vi "新记录通知-服务器版.vi"() -> ()   [LabVIEW 2013]
uses:
  <vilib>/Utility/miscctls.llb/LVRowAndColumnTypeDef.ctl
  <vilib>/Utility/inputDevices.llb/mouseAcquire.vi
panel:
  in  "列表菜单":enum16{"预览", "忽略此条", "删除缓存文件", "复制到剪贴板"}(ring)
  out "点到行列-实时列表":T1 caption="单元格位置"
  in  "device ID":refnum<k1> caption="设备ID"
  in  "新记录":cluster{"新记录列表行":string[], "对应缓存文件":string}[](array[cluster])
  in  "报警记录列表":i32[](listbox)
  in  "忽略全部":bool
  in  "预览全部":bool
  # "* 双击单元格打开预览\n  右键菜单中查看更多选项，管理界面中查看更多记录"
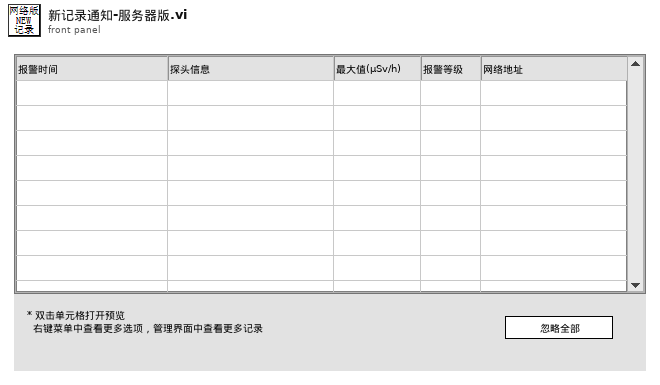
[diagram p1: front panel]
types:
  T1 = typedef "LVRowAndColumnTypeDef.ctl" = cluster{"Row":i32, "Column":i32}
  T2 = enum32{"Invalid", "Standard", "Closed", "Hidden", "Minimized", "Maximized"}
  T3 = typedef "LVPoint32TypeDef.ctl" = cluster{"Horizontal":i32, "Vertical":i32}
  T4 = cluster{"button 1":bool, "button 2":bool, "button 3":bool, "button 4":bool}
  T5 = cluster{"Shift":bool, "Ctrl":bool, "Alt":bool, "Cmd":bool, "Opt":bool}
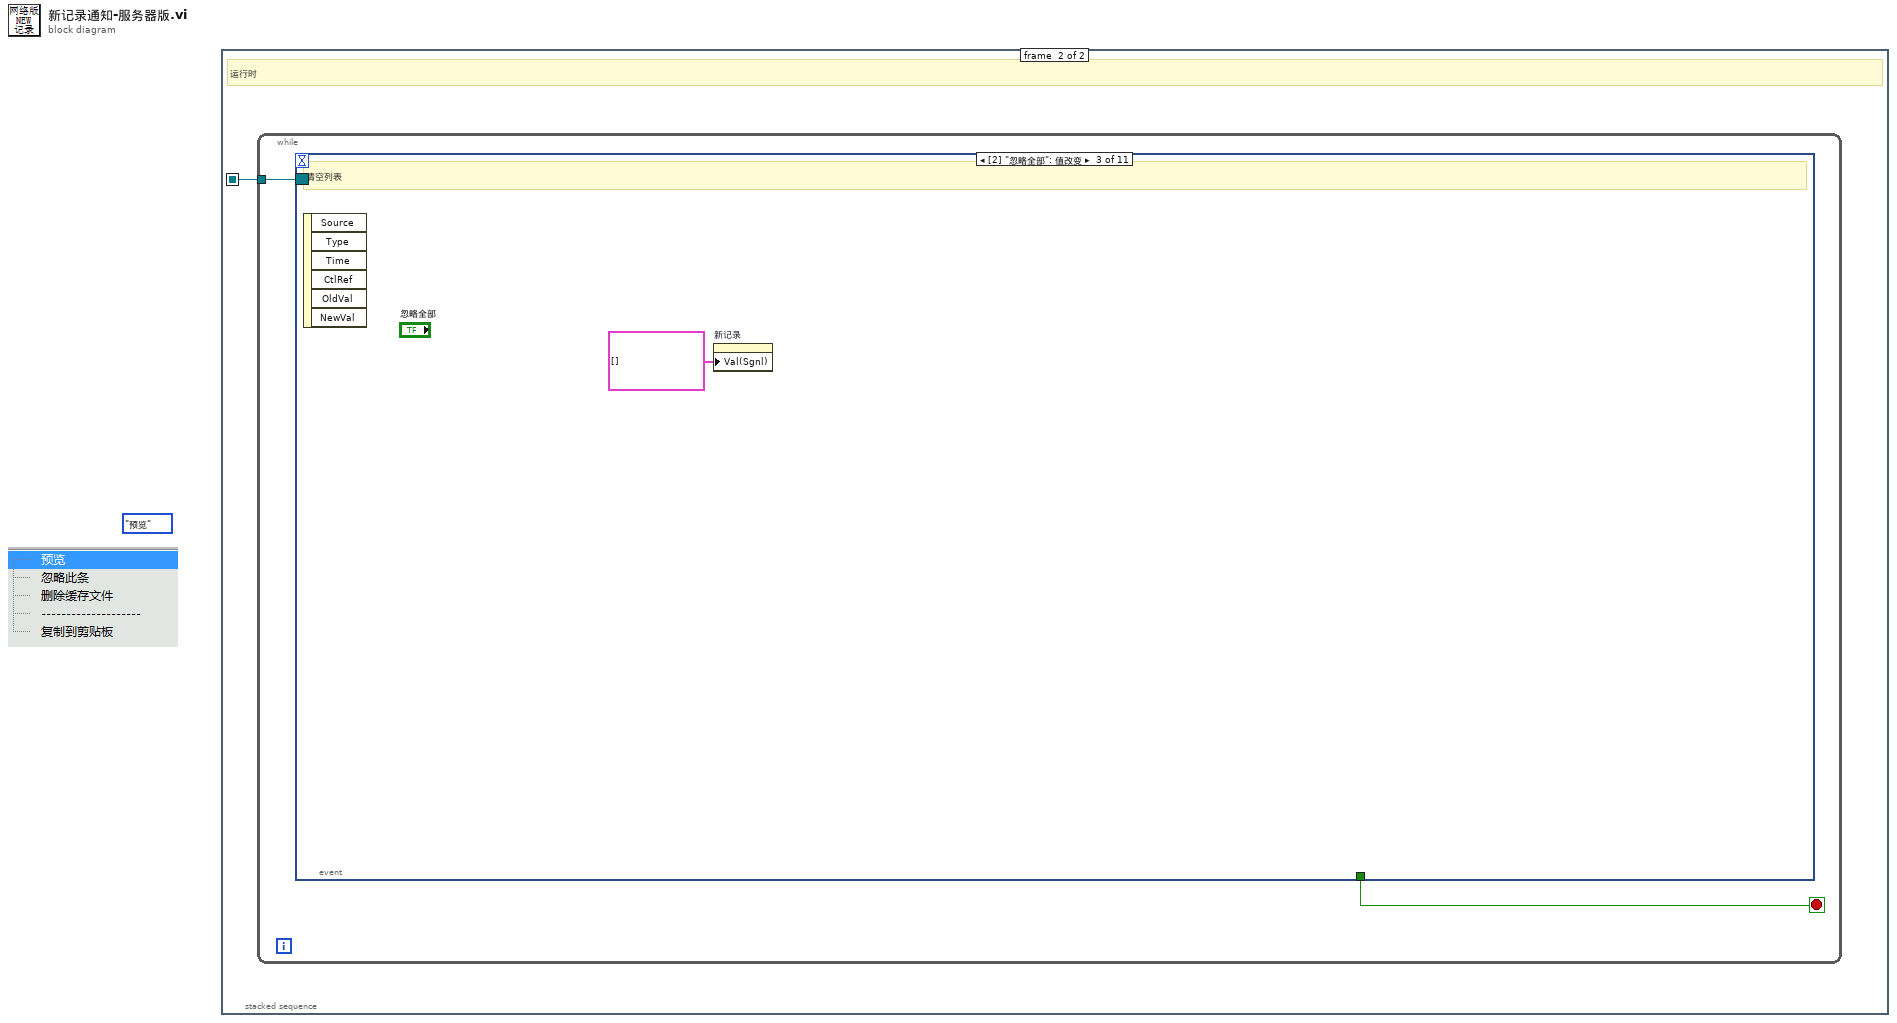
[diagram p0: block diagram]
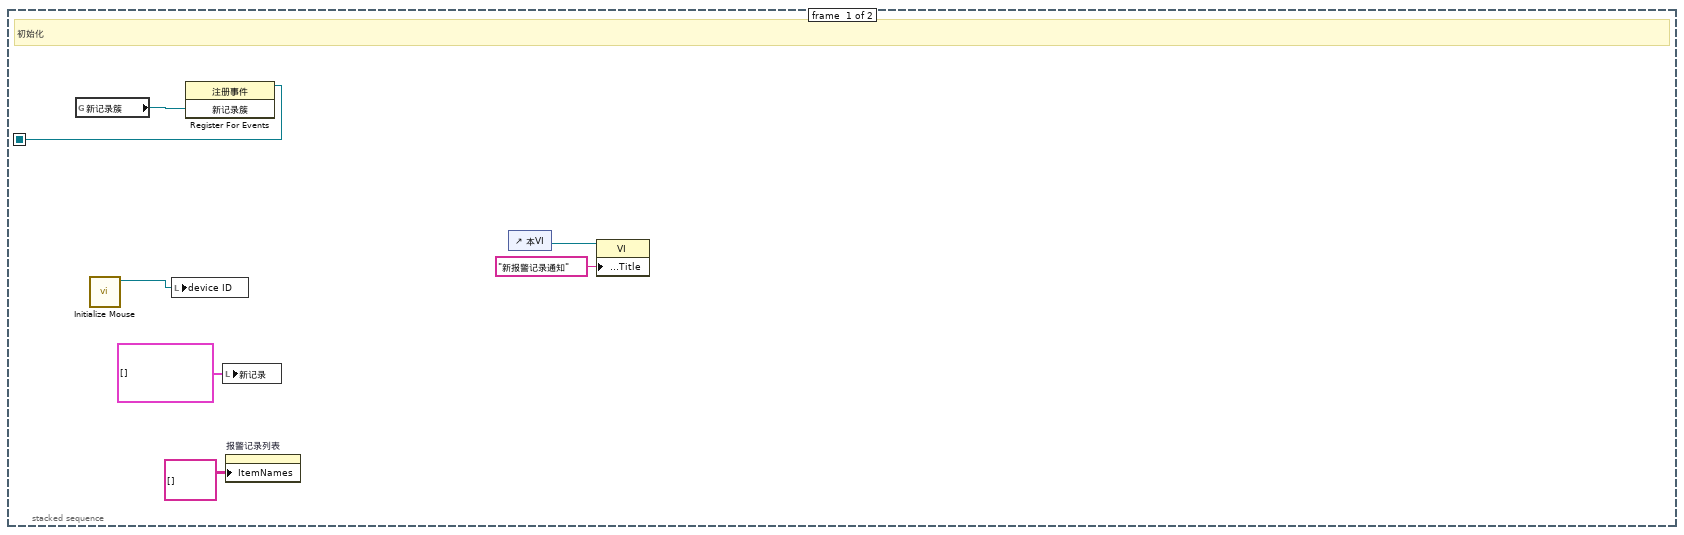
[diagram p2: hidden frame]
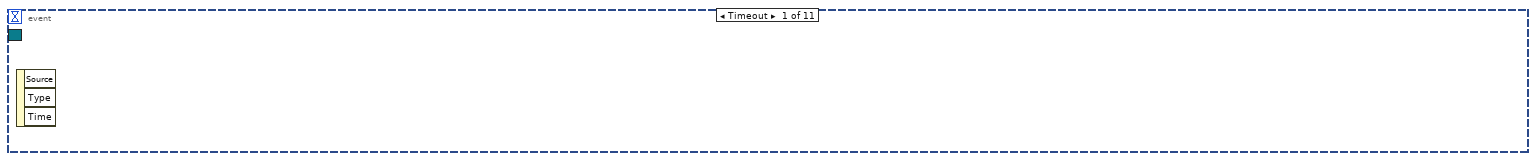
[diagram p3: hidden frame]
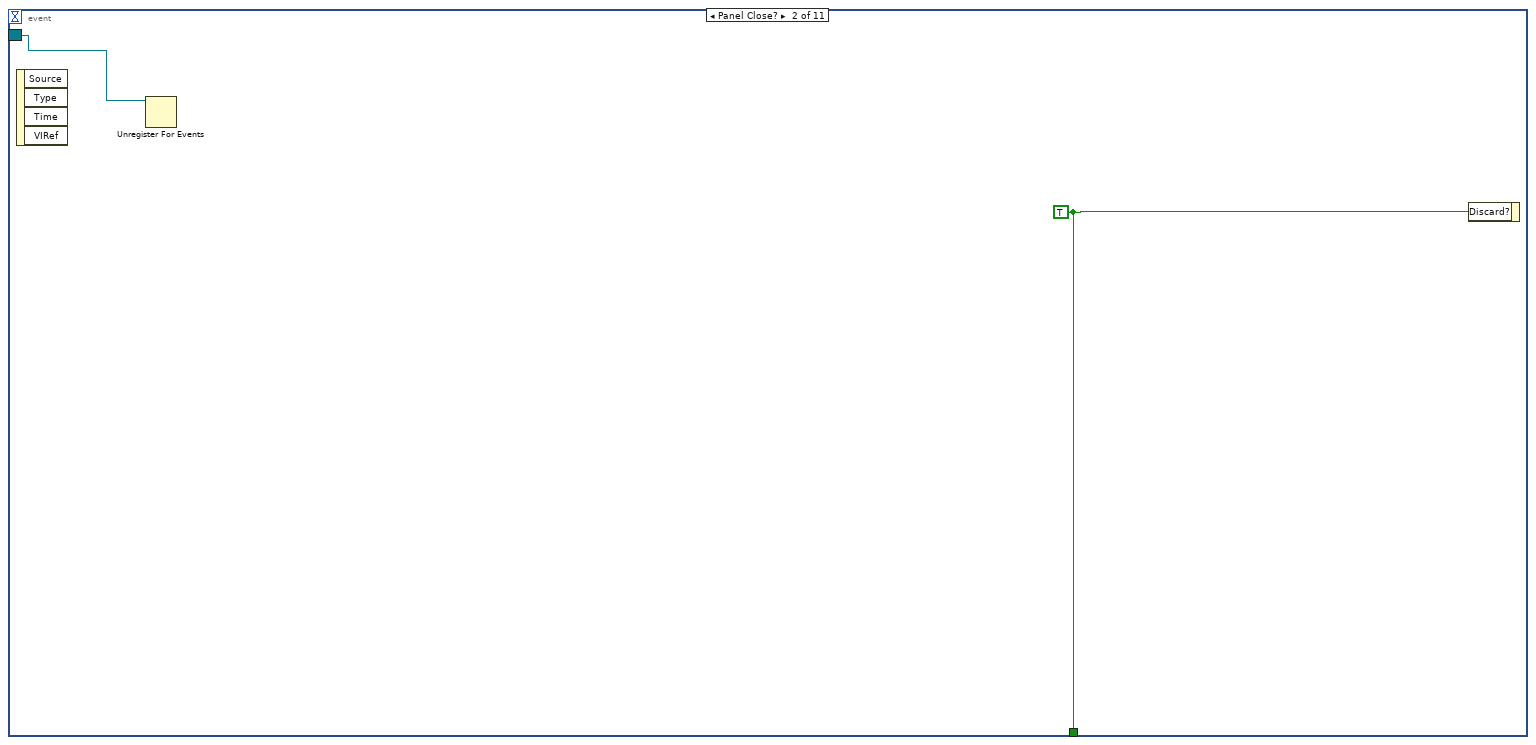
[diagram p4: hidden frame]
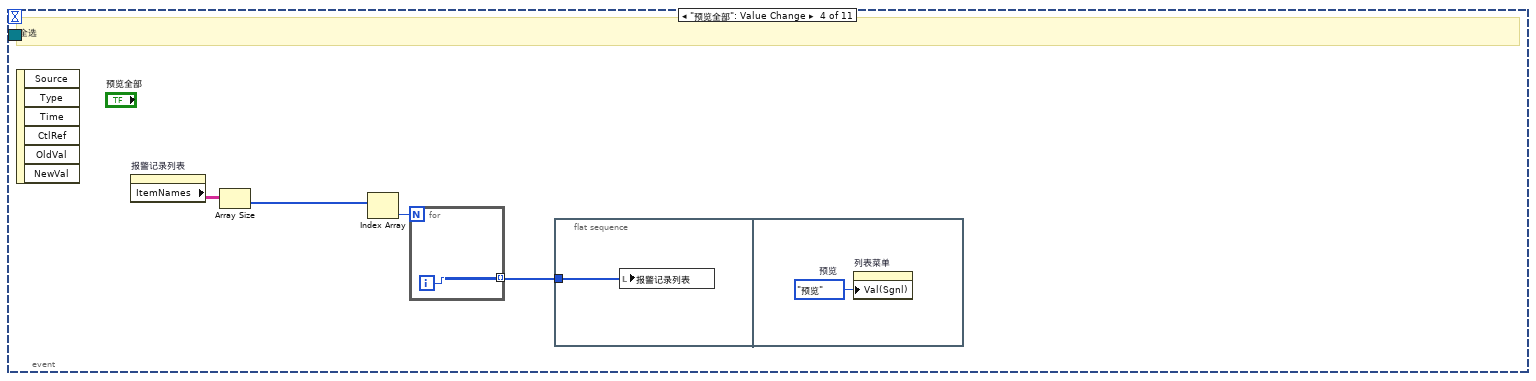
[diagram p5: hidden frame]
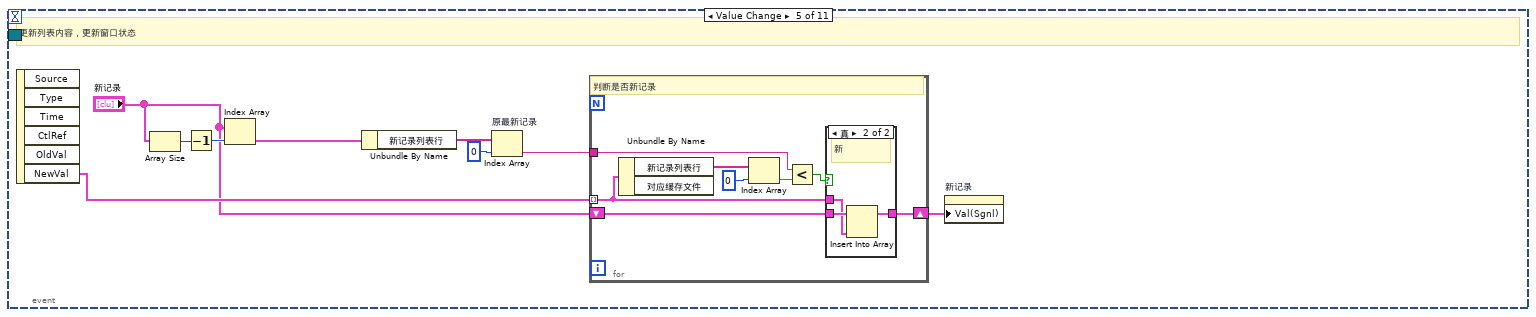
[diagram p6: hidden frame]
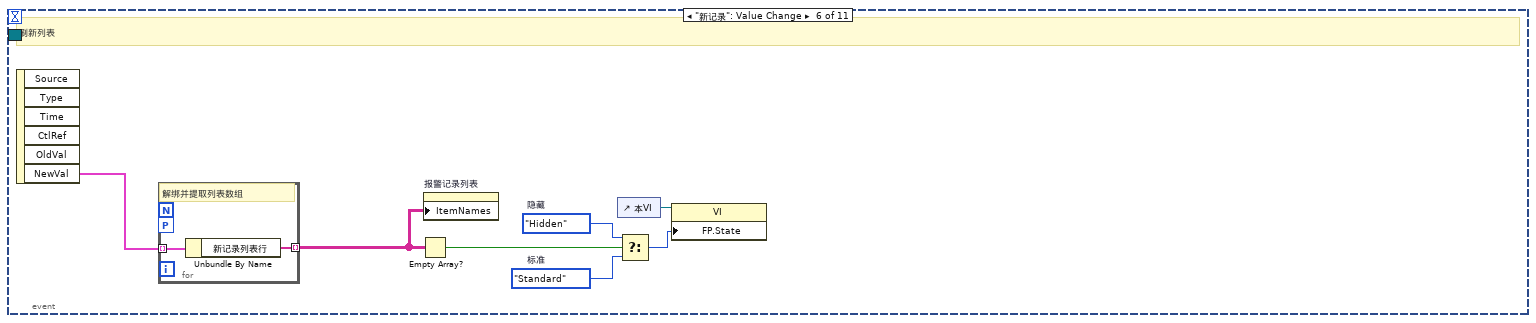
[diagram p8: hidden frame]
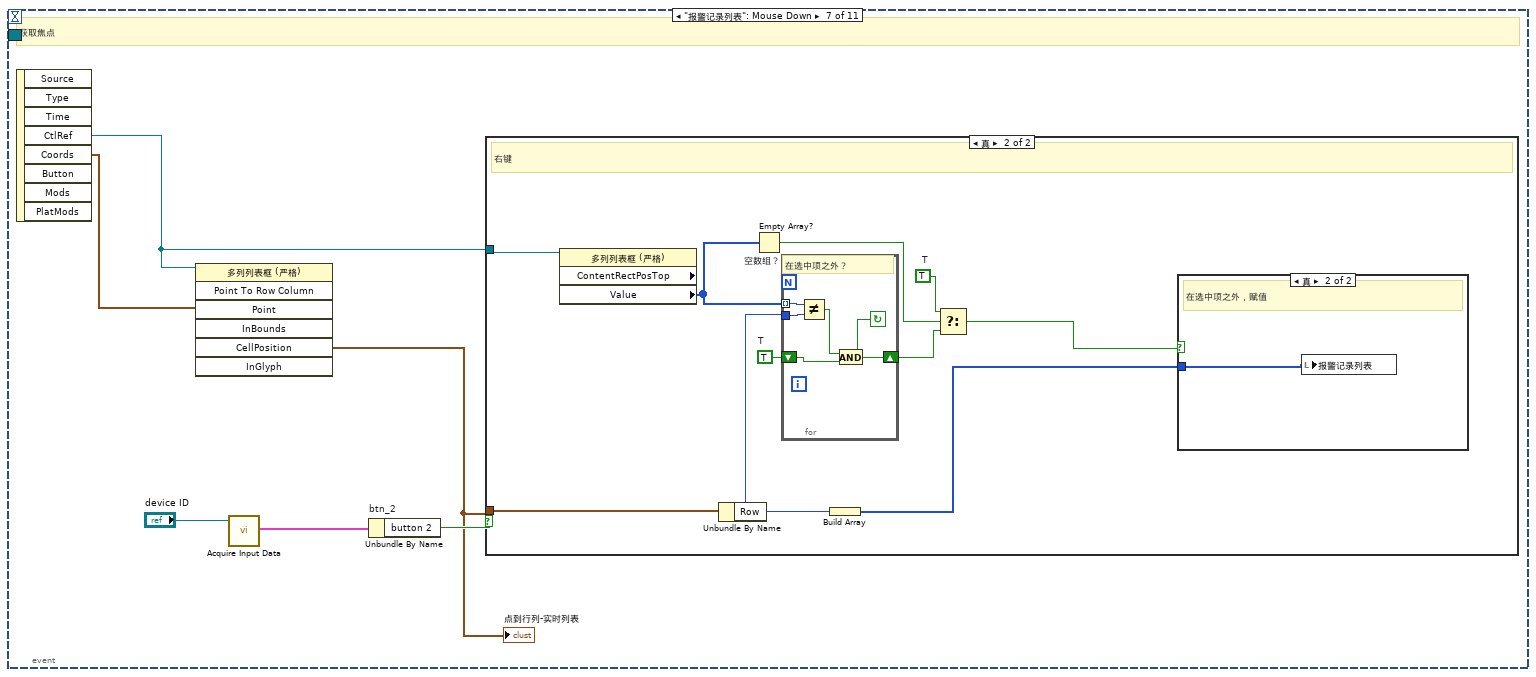
[diagram p9: hidden frame]
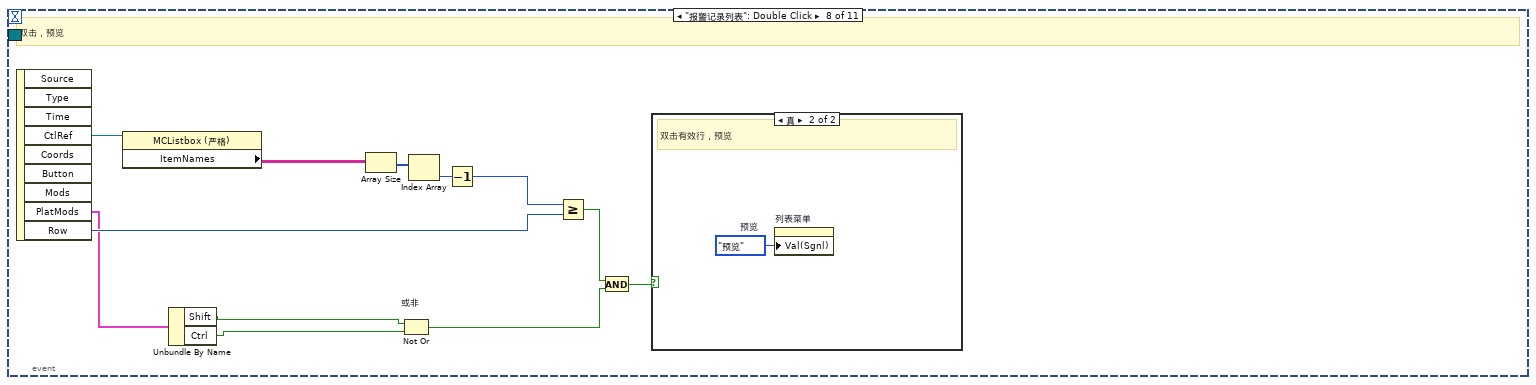
[diagram p12: hidden frame]
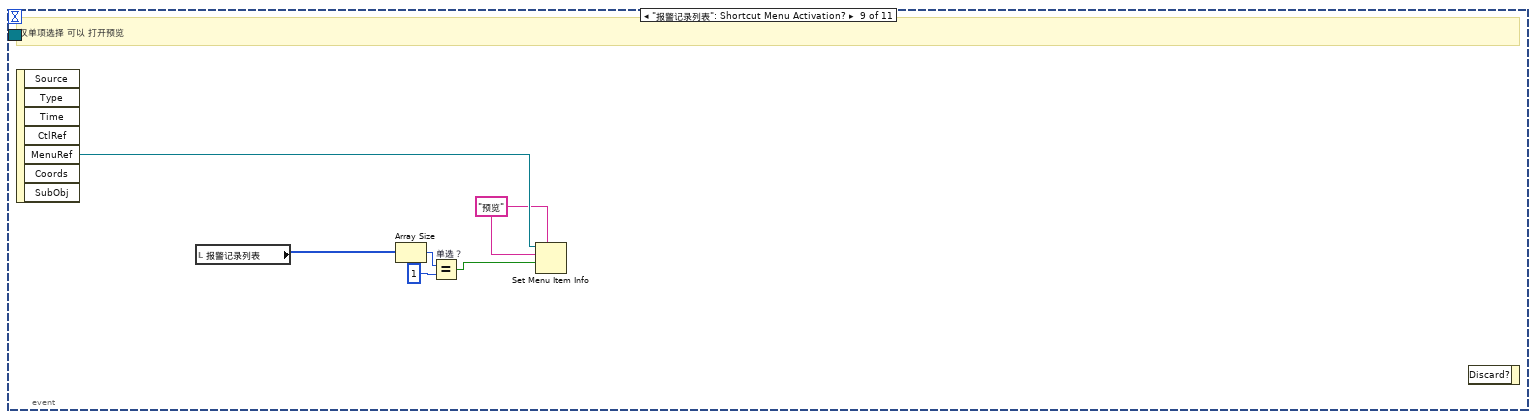
[diagram p14: hidden frame]
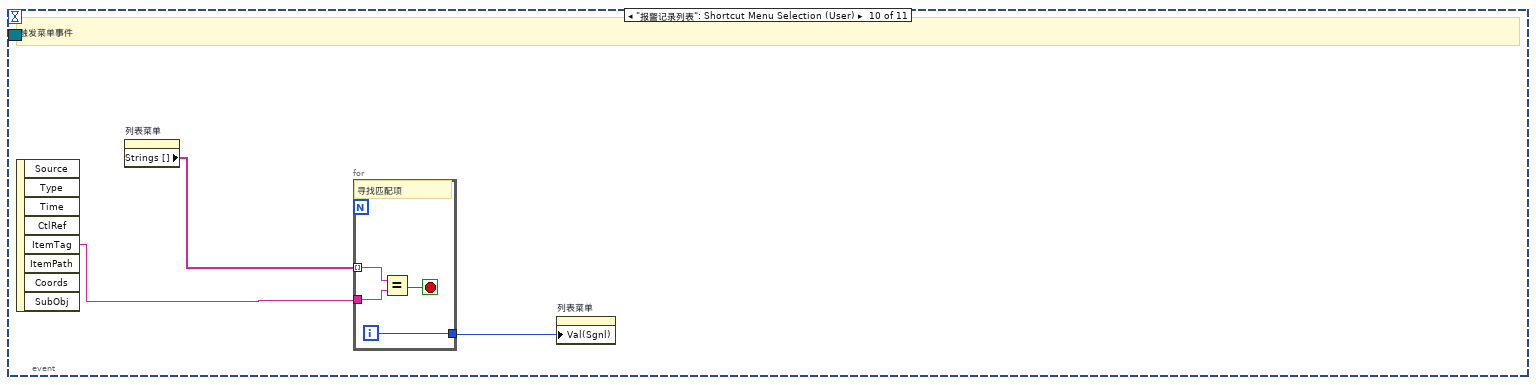
[diagram p15: hidden frame]
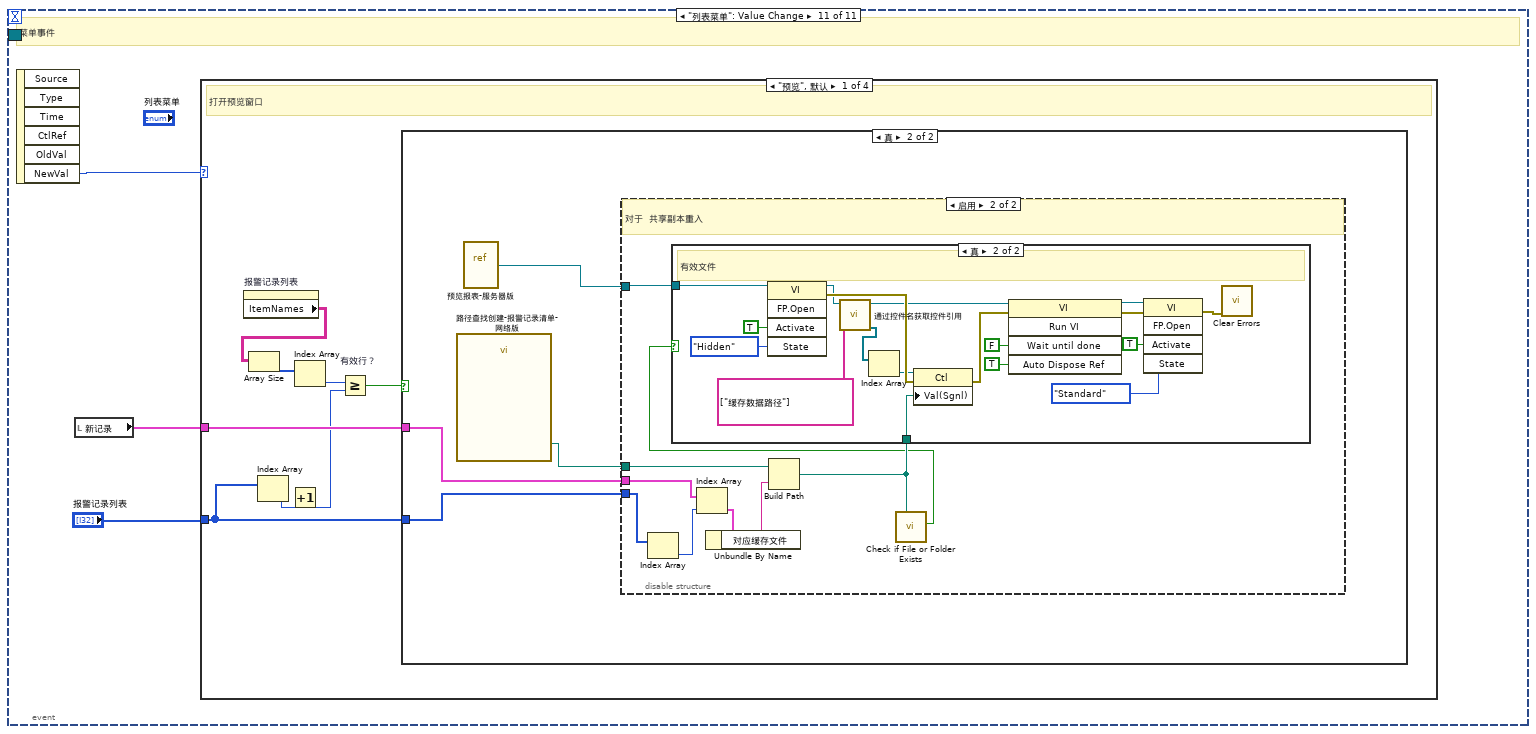
[diagram p16: hidden frame]
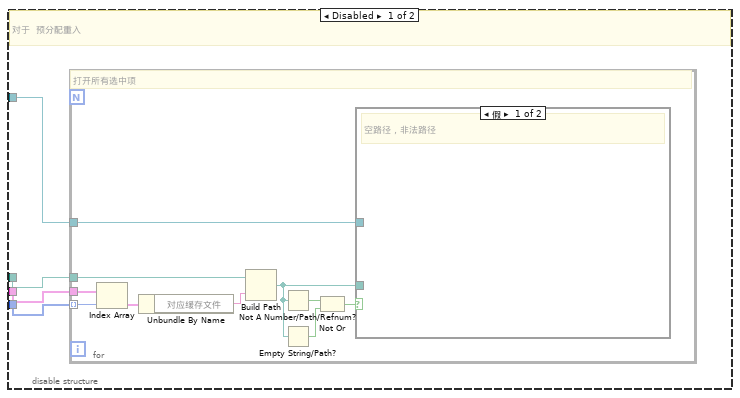
[diagram p18: hidden frame]
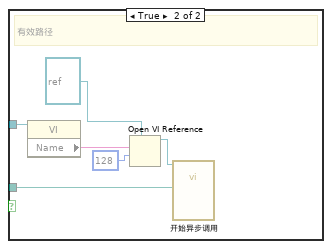
[diagram p19: hidden frame]
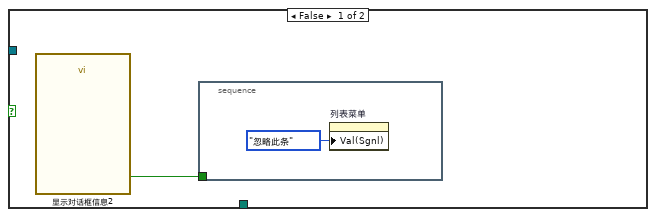
[diagram p20: hidden frame]
diagram:
  (unwired) enum16{"预览", "忽略此条", "删除缓存文件", "复制到剪贴板"}."预览"
  n1 = stacked-sequence {
    seq-local: [w6 _] -> [_ w8]
    frame #0 {
      # "初始化"
      n2 = global read "全局变量-35点监测.vi" "新记录簇"() -> (w7:refnum<vi>)
      n3 = call <vilib>:"Initialize Mouse.vi"() -> ("device ID"=w5:refnum<k1>)  [unwired: 10 in, 1 out]
      n4 = local write "device ID"(w5) -> ()
      n5 = register-events(w7) -> (reference out=w6:refnum<event-registration>)  [unwired: 2 in, 1 out]
      n6 = local write "新记录"(cluster{"新记录列表行":string[], "对应缓存文件":string}[] [] ("新记录")) -> ()
      n7 = property on="报警记录列表" class="MCListbox (严格)"("ItemNames"=string[][] [] ("项名")) -> ()  [unwired: 2 in, 2 out]
      n8 = control-ref of="本VI"() -> (w2:refnum<vi>)
      n9 = property class="VI"(reference=w2, "Front Panel.Title"="新报警记录通知" ("前面板窗口:标题")) -> ()  [unwired: 1 in, 2 out]
    }
    frame #1 {
      # "运行时"
      n10 = while {
        tunnel: w8 -> [w9]
        stop <- w10 stop-if-true
        n11 = event shown="[2] \"忽略全部\": 值改变" {
          selector: w9 -> [_ w11 _ _ _ _ _ _ _ _ _]
          dyn-events: _ -> [_ _ _ _ _ _ _ _ _ _ _]
          timeout: _ -> [_ _ _ _ _ _ _ _ _ _ _]
          tunnel: [_ w12 _ _ _ _ _ _ _ _ _] -> w10
          event Timeout {
            n12 = event-data() -> ()  [unwired: 1 in, 3 out]
          }
          event Panel Close? {
            w12 = TRUE ("放弃？")
            n13 = event-data() -> ()  [unwired: 1 in, 4 out]
            n14 = Unregister For Events(event registration refnum=w11) -> ()  [unwired: 1 in, 1 out]
            n15 = event-data("Discard?"=w12) -> ()  [unwired: 1 in, 1 out]
          }
          event "忽略全部": Value Change {
            # "清空列表"
            n16 = event-data() -> ()  [unwired: 1 in, 6 out]
            n17 = property on="新记录" class="Arr (严格)"("Val(Sgnl)"=cluster{"新记录列表行":string[], "对应缓存文件":string}[] [] ("值(信号)")) -> ()  [unwired: 2 in, 2 out]
          }
          event "预览全部": Value Change {
            # "全选"
            n18 = event-data() -> ()  [unwired: 1 in, 6 out]
            n19 = property on="报警记录列表" class="MCListbox (严格)"() -> ("ItemNames"=w17:string[][])  [unwired: 2 in, 2 out]
            n20 = Array Size(array=w17) -> (size(s)=w16:i32[])
            n21 = Index Array(array=w16) -> (element=w15:i32)  [unwired: 1 in]
            n22 = for {
              N: w15 -> [_]
              tunnel: [w18] -> w14 mode=indexing
              i -> [w18]
            }
            n23 = flat-sequence {
              tunnel: w14 -> [w19]
              frame #0 {
                n24 = local write "报警记录列表"(w19) -> ()
              }
              frame #1 {
                w20 = enum16{"预览", "忽略此条", "删除缓存文件", "复制到剪贴板"}."预览"  # 预览
                n25 = property on="列表菜单" class="Enum (严格)"("Val(Sgnl)"=w20) -> ()  [unwired: 2 in, 2 out]
              }
            }
          }
          event Value Change {
            # "更新列表内容，更新窗口状态"
            n26 = event-data() -> ("NewVal"=w28:cluster{"新记录列表行":string[], "对应缓存文件":string}[])  [unwired: 1 in, 5 out]
            n27 = Array Size(array="新记录") -> (size(s)=w27:i32)
            n28 = Decrement(x=w27) -> (x-1=w29:i32)
            n29 = Index Array(array="新记录", index=w29) -> (element=w26:cluster{"新记录列表行":string[], "对应缓存文件":string})
            n30 = Unbundle By Name(w26) -> ("新记录列表行"=w25:string[])
            n31 = Index Array "原最新记录"(array=w25, index=0 ("禁用的索引 (列)")) -> (element=w23:string)
            n32 = for {
              tunnel: w28 -> [w31] mode=indexing
              tunnel: w23 -> [w34]
              shift-right: [w30] -> w21
              shift-left: "新记录" -> [w32]
              # "判断是否新记录"
              n33 = Unbundle By Name(w31) -> ("新记录列表行"=w37:string[])  [unwired: 1 out]
              n34 = Index Array(array=w37, index=0 ("禁用的索引 (列)")) -> (element=w35:string)
              n35 = Less?(x=w34, y=w35) -> (x < y?=w33:bool)
              n36 = case shown="真" w33 {
                tunnel: w32 -> [w38 w41]
                tunnel: w31 -> [_ w40]
                tunnel: [w38 w39] -> w30
                frame False {
                  # "非新"
                }
                frame True {
                  # "新"
                  n37 = Insert Into Array(array=w41, new element=w40) -> (w39:cluster{"新记录列表行":string[], "对应缓存文件":string}[])  [unwired: 1 in]
                }
              }
            }
            n38 = property on="新记录" class="Arr (严格)"("Val(Sgnl)"=w21) -> ()  [unwired: 2 in, 2 out]
          }
          event "新记录": Value Change {
            w46 = T2."Hidden"  # 隐藏
            w45 = T2."Standard"  # 标准
            # "刷新列表"
            n39 = event-data() -> ("NewVal"=w48:cluster{"新记录列表行":string[], "对应缓存文件":string}[])  [unwired: 1 in, 5 out]
            n40 = for {
              workers-P: _ -> [_]
              tunnel: w48 -> [w50] mode=indexing
              tunnel: [w49] -> w43 mode=indexing
              # "解绑并提取列表数组"
              n41 = Unbundle By Name(w50) -> ("新记录列表行"=w49:string[])
            }
            n42 = Empty Array?(array=w43) -> (empty?=w42:bool)
            n43 = property on="报警记录列表" class="MCListbox (严格)"("ItemNames"=w43) -> ()  [unwired: 2 in, 2 out]
            n44 = control-ref of="本VI"() -> (w47:refnum<vi>)
            n45 = Select(t=w46, s=w42, f=w45) -> (s? t:f=w44:T2)
            n46 = property class="VI"(reference=w47, "FP.State"=w44) -> ()  [unwired: 1 in, 2 out]
          }
          event "报警记录列表": Mouse Down {
            # "获取焦点"
            n47 = event-data() -> ("CtlRef"=w52:refnum<vi>, "Coords"=w53:T3)  [unwired: 1 in, 6 out]
            n48 = invoke class="多列列表框 (严格)" method="Point To Row Column"(reference=w52, "Point"=w53) -> ("CellPosition"=w51:T1)  [unwired: 5 in, 6 out]
            "点到行列-实时列表" <- w51
            n49 = call-poly <vilib>:"Acquire Input Data.vi"("device ID"="device ID") -> ("button info"=w55:T4)  [unwired: 15 in, 3 out]
            n50 = Unbundle By Name "btn_2"(w55) -> ("button 2"=w56:bool)
            n51 = case shown="真" w56 {
              tunnel: w52 -> [_ w65]
              tunnel: w51 -> [_ w62]
              frame False {
                # "不是右键"
              }
              frame True {
                w59 = TRUE  # T
                w66 = TRUE  # T
                # "右键"
                n52 = property class="多列列表框 (严格)" props=["ContentRectPosTop", "Value"](reference=w65) -> ("Value"=w61:i32[])  [unwired: 1 in, 3 out]
                n53 = Unbundle By Name(w62) -> ("Row"=w64:i32)
                n54 = Empty Array? "空数组？"(array=w61) -> (empty?=w60:bool)
                n55 = for {
                  tunnel: w61 -> [w72] mode=indexing
                  shift-right: [w69] -> w58
                  shift-left: w66 -> [w70]
                  tunnel: w64 -> [w68]
                  stop <- w69 continue-if-true
                  # "在选中项之外？"
                  n56 = Not Equal?(x=w72, y=w68) -> (x != y?=w71:bool)
                  n57 = And(x=w71, y=w70) -> (x .and. y?=w69:bool)
                }
                n58 = Build Array(w64) -> (w63:i32[])
                n59 = Select(t=w59, s=w60, f=w58) -> (s? t:f=w57:bool)
                n60 = case shown="真" w57 {
                  tunnel: w63 -> [_ w67]
                  frame False {
                    # "在选中项之中，不赋值"
                  }
                  frame True {
                    # "在选中项之外，赋值"
                    n61 = local write "报警记录列表"(w67) -> ()
                  }
                }
              }
            }
          }
          event "报警记录列表": Double Click {
            # "双击，预览"
            n62 = event-data() -> ("CtlRef"=w84:refnum<vi>, "PlatMods"=w76:T5, "Row"=w79:i32)  [unwired: 1 in, 6 out]
            n63 = property class="MCListbox (严格)"(reference=w84) -> ("ItemNames"=w83:string[][])  [unwired: 1 in, 2 out]
            n64 = Unbundle By Name(w76) -> ("Shift"=w75:bool, "Ctrl"=w74:bool)
            n65 = Array Size(array=w83) -> (size(s)=w82:i32[])
            n66 = Not Or "或非"(1:w74, 2:w75) -> (0:w77:bool)
            n67 = Index Array(array=w82) -> (element=w81:i32)  [unwired: 1 in]
            n68 = Decrement(x=w81) -> (x-1=w80:i32)
            n69 = Greater Or Equal?(x=w80, y=w79) -> (x >= y?=w78:bool)
            n70 = And(x=w78, y=w77) -> (x .and. y?=w73:bool)
            n71 = case shown="真" w73 {
              frame False {
                # "无效行"
              }
              frame True {
                w85 = enum16{"预览", "忽略此条", "删除缓存文件", "复制到剪贴板"}."预览"  # 预览
                # "双击有效行，预览"
                n72 = property on="列表菜单" class="Enum (严格)"("Val(Sgnl)"=w85) -> ()  [unwired: 2 in, 2 out]
              }
            }
          }
          event "报警记录列表": Shortcut Menu Activation? {
            w87 = "预览" ("项标识符")
            # "仅单项选择 可以 打开预览"
            n73 = event-data() -> ("MenuRef"=w88:refnum<k9>)  [unwired: 1 in, 6 out]
            n74 = local read "报警记录列表"() -> (w91:i32[])
            n75 = Array Size(array=w91) -> (size(s)=w90:i32)
            n76 = Equal? "单选？"(x=w90, y=1) -> (x = y?=w86:bool)
            n77 = Set Menu Item Info(7:w87, 9:w86, 10:w87, 11:w88) -> ()  [unwired: 3 in, 2 out]
            n78 = event-data() -> ()  [unwired: 2 in, 1 out]
          }
          event "报警记录列表": Shortcut Menu Selection (User) {
            # "触发菜单事件"
            n79 = event-data() -> ("ItemTag"=w93:string)  [unwired: 1 in, 7 out]
            n80 = property on="列表菜单" class="Enum (严格)"() -> ("Strings []"=w94:string[])  [unwired: 2 in, 2 out]
            n81 = for {
              tunnel: w94 -> [w98] mode=indexing
              tunnel: w93 -> [w97]
              tunnel: [w95] -> w92
              i -> [w95]
              stop <- w96 stop-if-true
              # "寻找匹配项"
              n82 = Equal?(x=w98, y=w97) -> (x = y?=w96:bool)
            }
            n83 = property on="列表菜单" class="Enum (严格)"("Val(Sgnl)"=w92) -> ()  [unwired: 2 in, 2 out]
          }
          event "列表菜单": Value Change {
            # "菜单事件"
            n84 = event-data() -> ("NewVal"=w101:enum16{"预览", "忽略此条", "删除缓存文件", "复制到剪贴板"})  [unwired: 1 in, 5 out]
            n85 = local read "新记录"() -> (w99:cluster{"新记录列表行":string[], "对应缓存文件":string}[])
            n86 = case shown="\"预览\", 默认" w101 {
              tunnel: "报警记录列表" -> [w105 w166 w171 w196]
              tunnel: w99 -> [w109 w164 w172 _]
              frame "预览", Default {
                # "打开预览窗口"
                n87 = property on="报警记录列表" class="MCListbox (严格)"() -> ("ItemNames"=w106:string[][])  [unwired: 2 in, 2 out]
                n88 = Array Size(array=w106) -> (size(s)=w107:i32[])
                n89 = Index Array(array=w105) -> (element=w104:i32)  [unwired: 1 in]
                n90 = Increment(x=w104) -> (x+1=w103:i32)
                n91 = Index Array(array=w107) -> (element=w108:i32)  [unwired: 1 in]
                n92 = Greater Or Equal? "有效行？"(x=w108, y=w103) -> (x >= y?=w102:bool)
                n93 = case shown="真" w102 {
                  tunnel: w105 -> [_ w113]
                  tunnel: w109 -> [_ w112]
                  frame False {
                  }
                  frame True {
                    n94 = call "路径查找创建-报警记录清单-网络版.vi"() -> ("缓存数据文件夹"=w110:path)  [unwired: 1 in, 10 out]
                    n95 = vi-ref "预览报表-服务器版.vi"() -> (w111:refnum<vi>)
                    n96 = disable-structure shown="启用" {
                      disable-tunnel: w111 -> [w117 w136]
                      disable-tunnel: w110 -> [w116 w138]
                      disable-tunnel: w113 -> [w115 w141]
                      disable-tunnel: w112 -> [w114 w142]
                      frame Disabled {
                        # "对于  预分配重入"
                        n97 = for {
                          tunnel: w115 -> [w118] mode=indexing
                          tunnel: w117 -> [w127]
                          tunnel: w116 -> [w124]
                          tunnel: w114 -> [w126]
                          # "打开所有选中项"
                          n98 = Index Array(array=w126, index=w118) -> (element=w125:cluster{"新记录列表行":string[], "对应缓存文件":string})
                          n99 = Unbundle By Name(w125) -> ("对应缓存文件"=w123:string)
                          n100 = Build Path(base path=w124, name or relative path=w123) -> (appended path=w119:path)
                          n101 = Not A Number/Path/Refnum?(number/path/refnum=w119) -> (NaN/Path/Refnum?=w122:bool)
                          n102 = Empty String/Path?(string/path=w119) -> (empty?=w121:bool)
                          n103 = Not Or(1:w121, 2:w122) -> (0:w120:bool)
                          n104 = case shown="假" w120 {
                            tunnel: w127 -> [_ w129]
                            tunnel: w119 -> [_ w128]
                            frame False {
                              # "空路径，非法路径"
                            }
                            frame True {
                              # "有效路径"
                              n105 = property class="VI"(reference=w129) -> ("Name"=w131:string)  [unwired: 1 in, 2 out]
                              n106 = Open VI Reference(type specifier VI Refnum (for type only)=refnum<vi> refnum ("类型说明符VI引用句柄（仅用于类型）"), vi path=w131, options=128 ("选项")) -> (vi reference=w133:refnum<vi>)  [unwired: 3 in, 1 out]
                              n107 = call-by-ref "开始异步调用"(reference=w133, "缓存数据路径"=w128) -> ()  [unwired: 12 in, 2 out]
                            }
                          }
                        }
                      }
                      frame Enabled {
                        # "对于  共享副本重入"
                        n108 = Index Array(array=w141) -> (element=w140:i32)  [unwired: 1 in]
                        n109 = Index Array(array=w142, index=w140) -> (element=w139:cluster{"新记录列表行":string[], "对应缓存文件":string})
                        n110 = Unbundle By Name(w139) -> ("对应缓存文件"=w137:string)
                        n111 = Build Path(base path=w138, name or relative path=w137) -> (appended path=w135:path)
                        n112 = call <vilib>:"Check if File or Folder Exists.vi"("path"=w135) -> ("file or folder exists?"=w134:bool)  [unwired: 8 in, 2 out]
                        n113 = case shown="真" w134 {
                          tunnel: w136 -> [_ w146]
                          tunnel: w135 -> [_ w145]
                          frame False {
                            n114 = call "显示对话框信息2"() -> ("忽略此条"=w143:bool)  [unwired: 10 in, 1 out]
                            n115 = stacked-sequence {
                              tunnel: w143 -> [_]
                              frame #0 {
                                n116 = property on="列表菜单" class="Enum (严格)"("Val(Sgnl)"=enum16{"预览", "忽略此条", "删除缓存文件", "复制到剪贴板"}."忽略此条" ("值(信号)")) -> ()  [unwired: 2 in, 2 out]
                              }
                            }
                          }
                          frame True {
                            # "有效文件"
                            n117 = invoke class="VI" method="FP.Open"(reference=w146, "Activate"=TRUE ("激活？"), "State"=T2."Hidden" ("状态")) -> (reference out=w149:refnum<vi>, error out=w161:errorcluster)  [unwired: 2 in, 3 out]
                            n118 = call "通过控件名获取控件引用.vi"("控件名数组"=string[] ["缓存数据路径"], "VI引用"=w149) -> ("控件引用输出"=w151:refnum<vi>[], "VI引用o"=w153:refnum<vi>)  [unwired: 7 in, 1 out]
                            n119 = Index Array(array=w151) -> (element=w152:refnum<vi>)  [unwired: 1 in]
                            n120 = property class="Ctl"(reference=w152, error in=w161, "Val(Sgnl)"=w145) -> (error out=w162:errorcluster)  [unwired: 1 out]
                            n121 = invoke class="VI" method="Run VI"(reference=w153, error in=w162, "Wait until done"=FALSE ("结束前等待"), "Auto Dispose Ref"=TRUE ("自动销毁引用")) -> (reference out=w156:refnum<vi>, error out=w157:errorcluster)  [unwired: 1 in, 3 out]
                            n122 = invoke class="VI" method="FP.Open"(reference=w156, error in=w157, "Activate"=TRUE ("激活？"), "State"=T2."Standard" ("状态")) -> (error out=w160:errorcluster)  [unwired: 1 in, 4 out]
                            n123 = call <vilib>:"Clear Errors.vi"("error in (no error)"=w160) -> ()  [unwired: 6 in, 1 out]
                          }
                        }
                      }
                    }
                  }
                }
              }
              frame "忽略此条" {
                # "从“新记录”中删除，不删除缓存文件"
                n124 = Reverse 1D Array(array=w166) -> (reversed array=w165:i32[])
                n125 = for {
                  tunnel: w165 -> [w167] mode=indexing
                  shift-right: [w168] -> w163
                  shift-left: w164 -> [w169]
                  # "删除忽略项"
                  n126 = Delete From Array(array=w169, index=w167) -> (array with subset deleted=w168:cluster{"新记录列表行":string[], "对应缓存文件":string}[])  [unwired: 1 in, 1 out]
                }
                n127 = property on="新记录" class="Arr (严格)"("Val(Sgnl)"=w163) -> ()  [unwired: 2 in, 2 out]
              }
              frame "删除缓存文件" {
                # "删除缓存文件，刷新列表"
                n128 = call "显示对话框信息"() -> ("确定"=w170:bool)  [unwired: 10 in, 1 out]
                n129 = case shown="真" w170 {
                  tunnel: w172 -> [_ w174]
                  tunnel: w171 -> [_ w173]
                  frame False {
                    # "取消删除"
                  }
                  frame True {
                    # "确认删除"
                    n130 = stacked-sequence {
                      tunnel: w174 -> [w179 _]
                      tunnel: w173 -> [w178 _]
                      frame #0 {
                        # "删除文件，刷新列表"
                        n131 = call "路径查找创建-报警记录清单-网络版.vi"() -> ("缓存数据文件夹"=w175:path)  [unwired: 1 in, 10 out]
                        n132 = Reverse 1D Array(array=w178) -> (reversed array=w177:i32[])
                        n133 = for {
                          tunnel: w177 -> [w186] mode=indexing
                          shift-right: [w181] -> w176
                          shift-left: w179 -> [w187]
                          tunnel: w175 -> [w180]
                          # "删除文件与列表项"
                          n134 = Delete From Array(array=w187, index=w186) -> (deleted portion=w185:cluster{"新记录列表行":string[], "对应缓存文件":string}, array with subset deleted=w181:cluster{"新记录列表行":string[], "对应缓存文件":string}[])  [unwired: 1 in]
                          n135 = Unbundle By Name(w185) -> ("对应缓存文件"=w184:string)
                          n136 = Build Path(base path=w180, name or relative path=w184) -> (appended path=w182:path)
                          n137 = Delete(path (use dialog)=w182) -> (error out=w183:errorcluster)  [unwired: 4 in, 2 out]
                          n138 = call <vilib>:"Clear Errors.vi"("error in (no error)"=w183) -> ()  [unwired: 6 in, 1 out]
                        }
                        n139 = property on="新记录" class="Arr (严格)"("Val(Sgnl)"=w176) -> ()  [unwired: 2 in, 2 out]
                      }
                      frame #1 {
                        w188 = enum16{"刷新", "预览并生成报表", "删除记录", "复制选中项至剪贴板"}."刷新"  # 刷新
                        # "通知“管理VI”刷新报警记录列表"
                        n140 = vi-ref "多点监测上位机-服务器版.vi"() -> (w192:refnum<vi>)
                        n141 = call "通过控件名获取控件引用.vi"("控件名数组"=string[] ["菜单项-报警列表"], "VI引用"=w192) -> ("控件引用输出"=w190:refnum<vi>[])  [unwired: 7 in, 2 out]
                        n142 = Index Array(array=w190) -> (element=w189:refnum<vi>)  [unwired: 1 in]
                        n143 = property class="Ctl"(reference=w189, "Val(Sgnl)"=w188) -> ()  [unwired: 1 in, 2 out]
                      }
                    }
                  }
                }
              }
              frame "复制到剪贴板" {
                # "筛选选中项，到剪贴板"
                n144 = property on="报警记录列表" class="MCListbox (严格)"() -> ("ItemNames"=w197:string[][])  [unwired: 2 in, 2 out]
                n145 = for {
                  tunnel: w197 -> [w208]
                  tunnel: w196 -> [w206] mode=indexing
                  shift-right: [w204] -> w194
                  shift-left: string[][] [] ("ItemNames") -> [w207]
                  # "筛选选中项"
                  n146 = Index Array(array=w208, index (row)=w206) -> (element=w205:string[])  [unwired: 1 in]
                  n147 = Insert Into Array(array=w207, new element=w205) -> (w204:string[][])  [unwired: 2 in]
                }
                n148 = Array To Spreadsheet String(array=w194, 3:"%s" ("格式字符串")) -> (spreadsheet string=w201:string)  [unwired: 1 in]
                n149 = Array To Spreadsheet String(array=string[] ["报警时间", "探头信息", "最大值(μSv/h)", "报警等级", "网络地址"] ("ItemNames"), 3:"%s" ("格式字符串")) -> (spreadsheet string=w203:string)  [unwired: 1 in]
                n150 = control-ref of="本应用程序"() -> (w199:refnum<vi>)
                n151 = Concatenate Strings(w203, w201) -> (w202:string)
                n152 = invoke class="App" method="Clipboard.Write"(reference=w199, "Param 0"=w202) -> ()  [unwired: 2 in, 4 out]
              }
            }
          }
        }
      }
    }
  }
